vi "CAN Init.vi"(9 "pCanConfig":T1, 10 "CANIndex":u8, 11 "DevHandle":i32) -> (1 "pCanConfig out":T1, 3 "function return":i32)   [LabVIEW 2010, in "usb2can.lvlib"]
doc: "int WINAPI CAN_Init(int DevHandle, unsigned char CANIndex, CAN_INIT_CONFIG *pCanConfig);"
uses:
  usb2can.lvlib
  USB2XXX/trunk/USB2XXX/USB2XXX/vs2019/Release/USB2XXX.dll
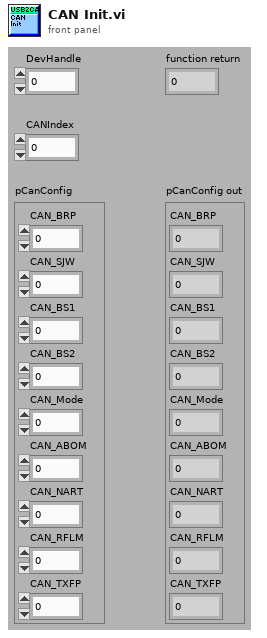
[diagram p1: front panel]
types:
  T1 = cluster{"CAN_BRP":u32, "CAN_SJW":u8, "CAN_BS1":u8, "CAN_BS2":u8, "CAN_Mode":u8, "CAN_ABOM":u8, "CAN_NART":u8, "CAN_RFLM":u8, "CAN_TXFP":u8}
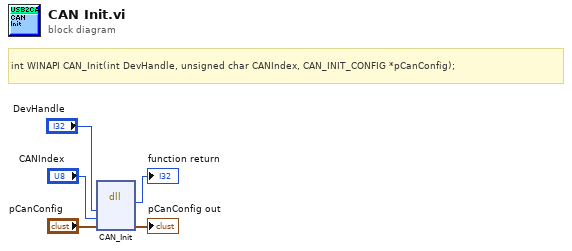
[diagram p0: block diagram]
diagram:
  # "int WINAPI CAN_Init(int DevHandle, unsigned char CANIndex, CAN_INIT_CONFIG *pCanConfig);"
  n1 = dll-call lib="E:/Projects/USB2XXX/trunk/USB2XXX/USB2XXX/vs2019/Release/USB2XXX.*" fn="CAN_Init"("DevHandle"="DevHandle", "CANIndex"="CANIndex", "pCanConfig"="pCanConfig") -> (→"function return":i32, "pCanConfig"=→"pCanConfig out":T1)  [unwired: 5 in, 2 out]
